vi "Laser wavelength change check.vi"(8 "error in (no error)":errorcluster, 11 "Laser 1 wavelength":dbl format="%#_13g") -> (0 "error out":errorcluster, 2 "Wavelength Out":u16, 3 "Proceed ?":bool)   [LabVIEW 2020]
uses:
  Global Variables/gl_UI Ctrl Refs.vi
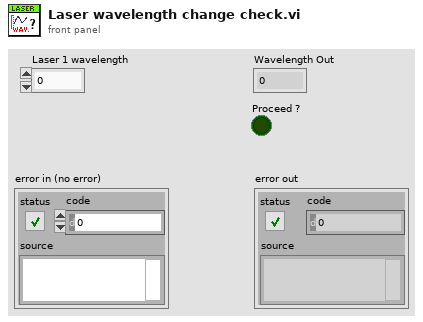
[diagram p1: front panel]
types:
  T1 = typedef "AOL_Globals.ctl" = cluster{"Imaging Protocol":T2, "Number of POI":u16, "Number of Miniscans":u16, "Number of Trials":u16, "Number of Cycles ":u64, "# Averaged Frames":u16, "Laser power (%)":u8, "Pockels (V)":dbl, "Acquisition Length (sec)":dbl, "Fill time (us)":dbl, "POI Dwell time (us)":dbl, "Miniscan Dwell time per pixel (us)":dbl, "PMT 1":dbl, "PMT 2":dbl, "Back Apperture (mA)":dbl, "Frame Size":T3, "Center Frequency":dbl, "Field of View (norm)":dbl, "DwellTime (us)":dbl, "Wavelength (nm)":dbl, "Zoom":dbl, "AOL Z":dbl, "AOL Mode":T4, "GridXY":dbl, "GridZ":dbl, "TriggerPeriod (sec)":dbl, "Number of Pixels in Miniscan":u16, "Experiment folder path":path, "X centre":dbl, "Y centre":dbl, "Angle (degrees)":dbl, "Plane Mode":T5, "Threshold":u16[], "Regenerate Chirps":bool, "Rectangle ROI length (pixels)":u16, "Rectangle ROI height (pixels)":u16, "AOD fill":u16, "StartupDelay":i32, "Samples Wait after Trigger":u16, "Slip Cycle":u32, "Add Cycle":bool, "Functional Mode":T6, "Z Start":dbl, "Z Stop":dbl, "# Planes":i32, "Total Pixels":i32, "Variable Miniscan Pixels":u16[], "Use Variable Length":bool, "Use Variable Resolution":bool, "Laser power (%) at Z Start":u8, "Laser power (%) at Z Stop":u8, "Ref Z Step":i8, "Ref Dwell Time (us)":dbl, "Field of View (um)":dbl}
  T2 = typedef "Imaging Protocols enum.ctl" = enum16{"AOL Z-Stack", "Motor Z Stack", "Functional Acquisition", "Single Plane Acquisition", "Volume Acquisition", "Live Imaging", "Live Plane Imaging", "Live Volume Imaging"}
  T3 = typedef "Frame Size.ctl" = u16
  T4 = typedef "AOL modes.ctl" = enum16{"Raster", "Structural", "Pointing", "Mini Scan", "Alignment"}
  T5 = typedef "Plane Mode.ctl" = u16
  T6 = typedef "Functional Mode.ctl" = enum16{"Point", "Line", "Patch", "Plane", "Volume"}
  T7 = typedef "UI ctrl refs cluster.ctl" = cluster{"Top level VI path":path, "Top level VI ref":refnum<vi>, "User menu ref":refnum<k9>, "Sub Panel control":refnum<vi>, "Imaging Param Tab":refnum<vi>, "Occurrence-Start drivers":refnum<k4>, "Occurrence-Speed logging initialised":refnum<k4>, "Occurrence-XYZ stage initialised":refnum<k4>, "Exit button":refnum<vi>, "Status ind":refnum<vi>, "Set as origin":refnum<vi>, "Speed Logging":refnum<vi>, "Time Lapse":refnum<vi>, "Live Imaging":refnum<vi>, "AOL Z Stack":refnum<vi>, "Motor Z Stack":refnum<vi>, "Funct Acq button":refnum<vi>, "Hard Shutter":refnum<vi>, "Virtual Shutter":refnum<vi>, "Laser Power":refnum<vi>, "AOL Mode":refnum<vi>, "Frame Size":refnum<vi>, "Field of View":refnum<vi>, "Dwell Time":refnum<vi>, "Zoom":refnum<vi>, "AOL Z":refnum<vi>, "Objective":refnum<vi>, "Axis":refnum<vi>, "Paths & Names":refnum<vi>, "Experiment folder path (ind.)":refnum<vi>, "Last State (Ind.)":refnum<vi>, "Averages":refnum<vi>, "Angle (degrees)":refnum<vi>, "X centre":refnum<vi>, "Y centre":refnum<vi>, "Plane Mode":refnum<vi>, "# Planes":refnum<vi>, "Z Start":refnum<vi>, "Z Stop":refnum<vi>, "Z Step":refnum<vi>, "PMT 1":refnum<vi>, "PMT 2":refnum<vi>, "Stage XYZ Position":refnum<vi>, "Pockels@Z Start":refnum<vi>, "Pockels@Z Stop":refnum<vi>, "Obtain Z Start":refnum<vi>, "Obtain Z Stop":refnum<vi>, "Live stim.trig.period":refnum<vi>, "Live stim.trig.enable":refnum<vi>, "Movement Correction":refnum<vi>, "Load Reference Image":refnum<vi>, "XY Stage Move":refnum<vi>, "MovCor Cluster":refnum<vi>, "RefDAQParam":refnum<vi>, "Funct. Acq. Pockels Modulation":refnum<vi>, "Ref Laser Power":refnum<vi>, "Enable Video Recording":refnum<vi>, "Video Record-Live Imaging":refnum<vi>, "Video Record-Funct acq":refnum<vi>, "Reference Source":refnum<vi>, "AOL Z-stack Chirps Ready (ind)":refnum<vi>, "Target time between mov.cor. ref triggers (ms)":refnum<vi>, "Funct. Acq. Ref frame save":refnum<vi>, "Tracking button":refnum<vi>, "Show ref plots window":refnum<vi>, "Center freq ind (nm)":refnum<vi>, "Pickup mode (ind)":refnum<vi>, "Logging queue (ind)":refnum<vi>, "Back aperture power (ind.)":refnum<vi>, "Power after objective (ind.)":refnum<vi>, "Switch user":refnum<vi>, "Ls1 Conn. Status":refnum<vi>, "Ls1Tuning Status":refnum<vi>, "Ls1 Faults":refnum<vi>, "Ls1 Connection":refnum<vi>, "Ls1 Mode":refnum<vi>, "Ls1 POWER [mW]":refnum<vi>, "Ls1Shutter":refnum<vi>, "Ls1 Wavelength":refnum<vi>, "Ls1 Note":refnum<vi>, "Ls1 Confirm Wav":refnum<vi>, "Ls1 PreChrp Prism1":refnum<vi>, "Ls1 PreChrp Prism2":refnum<vi>, "Ls1 wav top Ind":refnum<vi>, "Ls1 power top Ind":refnum<vi>, "Ls1 Pump peak Hold":refnum<vi>, "Ls1 Status Ind":refnum<vi>, "Ls1 wav cancel":refnum<vi>, "Experiment Type":refnum<vi>, "Biology Information":refnum<vi>, "Camera recording status":refnum<vi>}
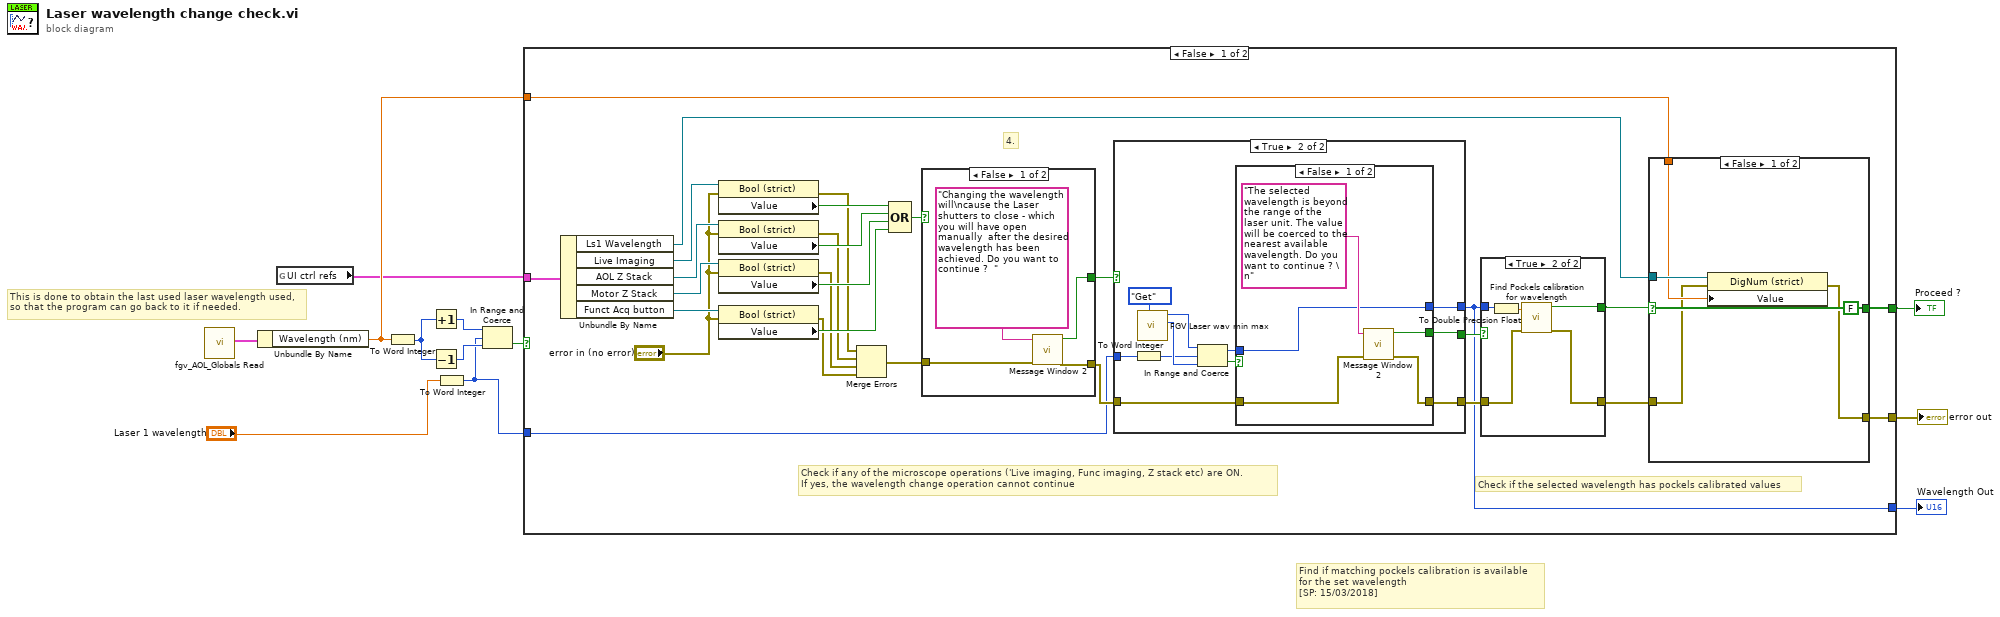
[diagram p0: block diagram]
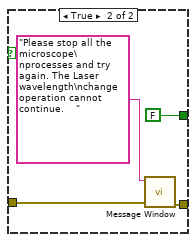
[diagram p6: hidden frame]
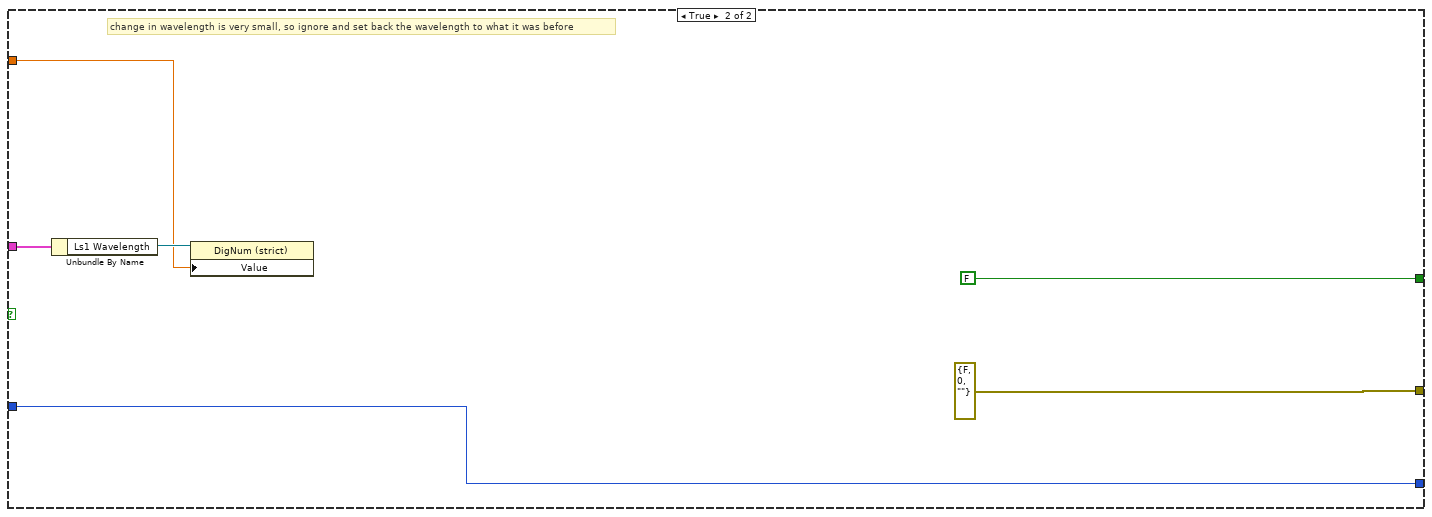
[diagram p7: hidden frame]
diagram:
  # "Find if matching pockels calibration is available \nfor the set wavelength\n[SP: 15/03/2018]"
  # "This is done to obtain the last used laser wavelength used,\nso that the program can go back to it if needed."
  n1 = call "fgv_AOL_Globals Read.vi"() -> ("AOL_Globals"=w9:T1)  [unwired: 9 in, 2 out]
  n2 = Unbundle By Name(w9) -> ("Wavelength (nm)"=w3:dbl)
  n3 = global read "gl_UI Ctrl Refs.vi" "UI ctrl refs"() -> (w1:T7)
  n4 = To Word Integer(number=w3) -> (16bit integer=w7:i16)
  n5 = Increment(x=w7) -> (x+1=w6:i16)
  n6 = Decrement(x=w7) -> (x-1=w5:i16)
  n7 = To Word Integer(number="Laser 1 wavelength") -> (16bit integer=w2:i16)
  n8 = In Range and Coerce(upper limit=w6, x=w2, lower limit=w5) -> (In Range?=w4:bool)  [unwired: 1 out]
  n9 = case shown="False" w4 {
    tunnel: [w23 FALSE] -> w12
    tunnel: [w22 errorcluster {"status"=FALSE, "code"=0, "source"=""} ("error out (no error)")] -> w11
    tunnel: [w17 w86] -> w10
    tunnel: w3 -> [w15 w88]
    tunnel: w1 -> [w14 w90]
    tunnel: w2 -> [w13 w86]
    frame False {
      # "4."
      # "Check if the selected wavelength has pockels calibrated values"
      # "Check if any of the microscope operations ('Live imaging, Func imaging, Z stack etc) are ON.\nIf yes, the wavelength change operation cannot continue"
      n10 = Unbundle By Name(w14) -> ("Ls1 Wavelength"=w16:refnum<vi>, "Live Imaging"=w40:refnum<vi>, "AOL Z Stack"=w39:refnum<vi>, "Motor Z Stack"=w38:refnum<vi>, "Funct Acq button"=w37:refnum<vi>)
      n11 = property class="Bool (strict)"(reference=w40, error in="error in (no error)") -> (error out=w30:errorcluster, "Value"=w36:bool)  [unwired: 1 out]
      n12 = property class="Bool (strict)"(reference=w39, error in="error in (no error)") -> (error out=w29:errorcluster, "Value"=w35:bool)  [unwired: 1 out]
      n13 = property class="Bool (strict)"(reference=w38, error in="error in (no error)") -> (error out=w28:errorcluster, "Value"=w34:bool)  [unwired: 1 out]
      n14 = property class="Bool (strict)"(reference=w37, error in="error in (no error)") -> (error out=w27:errorcluster, "Value"=w33:bool)  [unwired: 1 out]
      n15 = Merge Errors(w30, w29, w28, w27) -> (w26:errorcluster)
      n16 = Compound Arithmetic op=OR(w36, w35, w34, w33) -> (w32:bool)
      n17 = case shown="False" w32 {
        tunnel: w26 -> [w80 w84]
        tunnel: [w79 w83] -> w20
        tunnel: [w77 FALSE] -> w21
        frame False {
          n18 = call "Message Window 2.vi"("error in (no error)"=w80, "Message string"="Changing the wavelength will\ncause the Laser shutters to close - which you will have open manually  after the desired wavelength has been achieved. Do you want to continue ?  ") -> ("error out (no error)"=w79:errorcluster, "Ok ?"=w77:bool)  [unwired: 8 in]
        }
        frame True {
          n19 = call "Message Window.vi"("error in (no error)"=w84, "Message string"="Please stop all the microscope\nprocesses and try again. The Laser wavelength\nchange operation cannot continue.    ") -> ("error out (no error)"=w83:errorcluster)  [unwired: 9 in]
        }
      }
      n20 = case shown="True" w21 {
        selector: w21 -> [w43 _]
        tunnel: w20 -> [w42 w47]
        tunnel: [w42 w46] -> w19
        tunnel: w13 -> [w41 w50]
        tunnel: [w43 w45] -> w18
        tunnel: [w41 w44] -> w17
        frame False {
        }
        frame True {
          n21 = To Word Integer(number=w50) -> (16bit integer=w51:i16)
          n22 = call "FGV Laser wav min max.vi"("FGV Actions"=enum16{"Get", "Set"}."Get") -> ("Tmin Out"=w54:u16, "Tmax Out"=w53:u16)  [unwired: 8 in, 1 out]
          n23 = In Range and Coerce(upper limit=w53, x=w51, lower limit=w54) -> (coerced(x)=w48:u16, In Range?=w49:bool)
          n24 = case shown="False" w49 {
            selector: w49 -> [_ w60]
            tunnel: w48 -> [w55 w61]
            tunnel: w47 -> [w59 w62]
            tunnel: [w58 w62] -> w46
            tunnel: [w56 w60] -> w45
            tunnel: [w55 w61] -> w44
            frame False {
              n25 = call "Message Window 2.vi"("error in (no error)"=w59, "Message string"="The selected wavelength is beyond the range of the laser unit. The value will be coerced to the nearest available wavelength. Do you want to continue ? \n") -> ("error out (no error)"=w58:errorcluster, "Ok ?"=w56:bool)  [unwired: 8 in]
            }
            frame True {
            }
          }
        }
      }
      n26 = case shown="True" w18 {
        selector: w18 -> [w70 _]
        tunnel: w19 -> [w71 w75]
        tunnel: [w71 w74] -> w24
        tunnel: [w70 w76] -> w25
        tunnel: w17 -> [_ w73]
        frame False {
        }
        frame True {
          n27 = To Double Precision Float(number=w73) -> (double precision float=w72:dbl)
          n28 = call "Find Pockels calibration for wavelength.vi"("error in (no error)"=w75, "Wav"=w72) -> ("error out"=w74:errorcluster, "Ok ?"=w76:bool)  [unwired: 8 in]
        }
      }
      n29 = case shown="False" w25 {
        selector: w25 -> [_ w69]
        tunnel: w24 -> [w65 w68]
        tunnel: [FALSE w69] -> w23
        tunnel: [w64 w68] -> w22
        tunnel: w15 -> [w66 _]
        tunnel: w16 -> [w67 _]
        frame False {
          n30 = property class="DigNum (strict)"(reference=w67, error in=w65, "Value"=w66) -> (error out=w64:errorcluster)  [unwired: 1 out]
        }
        frame True {
        }
      }
    }
    frame True {
      # "change in wavelength is very small, so ignore and set back the wavelength to what it was before"
      n31 = Unbundle By Name(w90) -> ("Ls1 Wavelength"=w89:refnum<vi>)
      n32 = property class="DigNum (strict)"(reference=w89, "Value"=w88) -> ()  [unwired: 1 in, 2 out]
    }
  }
  "error out" <- w11
  "Proceed ?" <- w12
  "Wavelength Out" <- w10
